vi "InterDataCommunication_ZA.vi"(8 "error in (no error)":errorcluster, 10 "InterDataCommunication_ZA":T1={"State Name"="Init", "Data"=variant}, 11 "Zen Analytics in":refnum<class "Zen Analytics.lvclass">) -> (0 "error out":errorcluster, 3 "Zen Analytics out":refnum<class "Zen Analytics.lvclass">)   [LabVIEW 2019, in "Zen Analytics.lvlib" / "Zen Analytics.lvclass"]
uses:
  Zen Analytics.lvclass
  Dependency/InterDataCommunication.ctl
types:
  T1 = typedef "Zen Analytics.lvlib/Zen Analytics.lvclass/InterDataCommunication.ctl" = cluster{"State Name":string, "Data":variant}
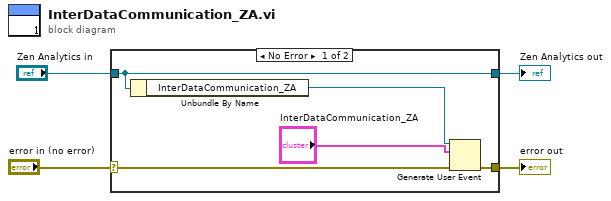
[diagram p0: block diagram]
diagram:
  n1 = case shown="No Error" "error in (no error)" {
    selector: "error in (no error)" -> [w7 w11]
    tunnel: [w6 w11] -> w3
    tunnel: [w9 w10] -> w1
    tunnel: "Zen Analytics in" -> [w9 w10]
    frame No Error {
      n2 = Unbundle By Name(w9) -> ("InterDataCommunication_ZA"=w8:refnum<user-event>)
      n3 = Generate User Event(user event=w8, event data cluster="InterDataCommunication_ZA", error in=w7) -> (error out=w6:errorcluster)  [unwired: 1 in, 1 out]
    }
    frame Error {
    }
  }
  "error out" <- w3
  "Zen Analytics out" <- w1
